vi "Temperature read hard mode 2.vi"() -> ()   [LabVIEW 2020]
panel:
  in  "START/STOP 2":bool
  out "START/STOP":bool
  in  "STOP":bool
  out "Waveform Chart":T1(graph)
  out "WARNING":bool
  in  "Filename":path
  in  "LOW Limit":dbl(slide) scale=0.0..100.0
  in  "C   or   F":bool
  in  "HIGH Limit":dbl(slide) scale=0.0..100.0
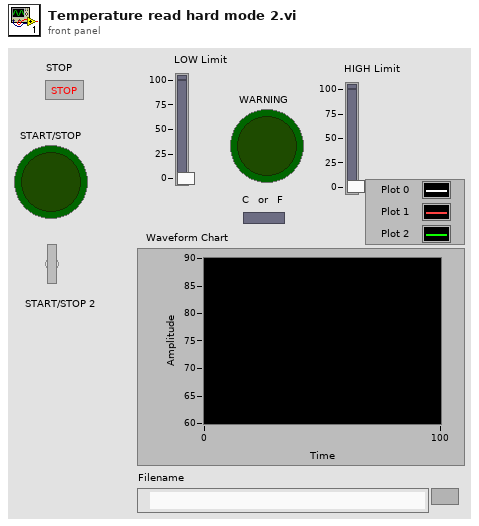
[diagram p1: front panel]
types:
  T1 = cluster{"Temperature (deg F)":dbl, "LOW Limit":dbl, "HIGH Limit":dbl}
  T2 = enum16{"open", "replace", "create", "open or create", "replace or create", "replace or create with confirmation"}
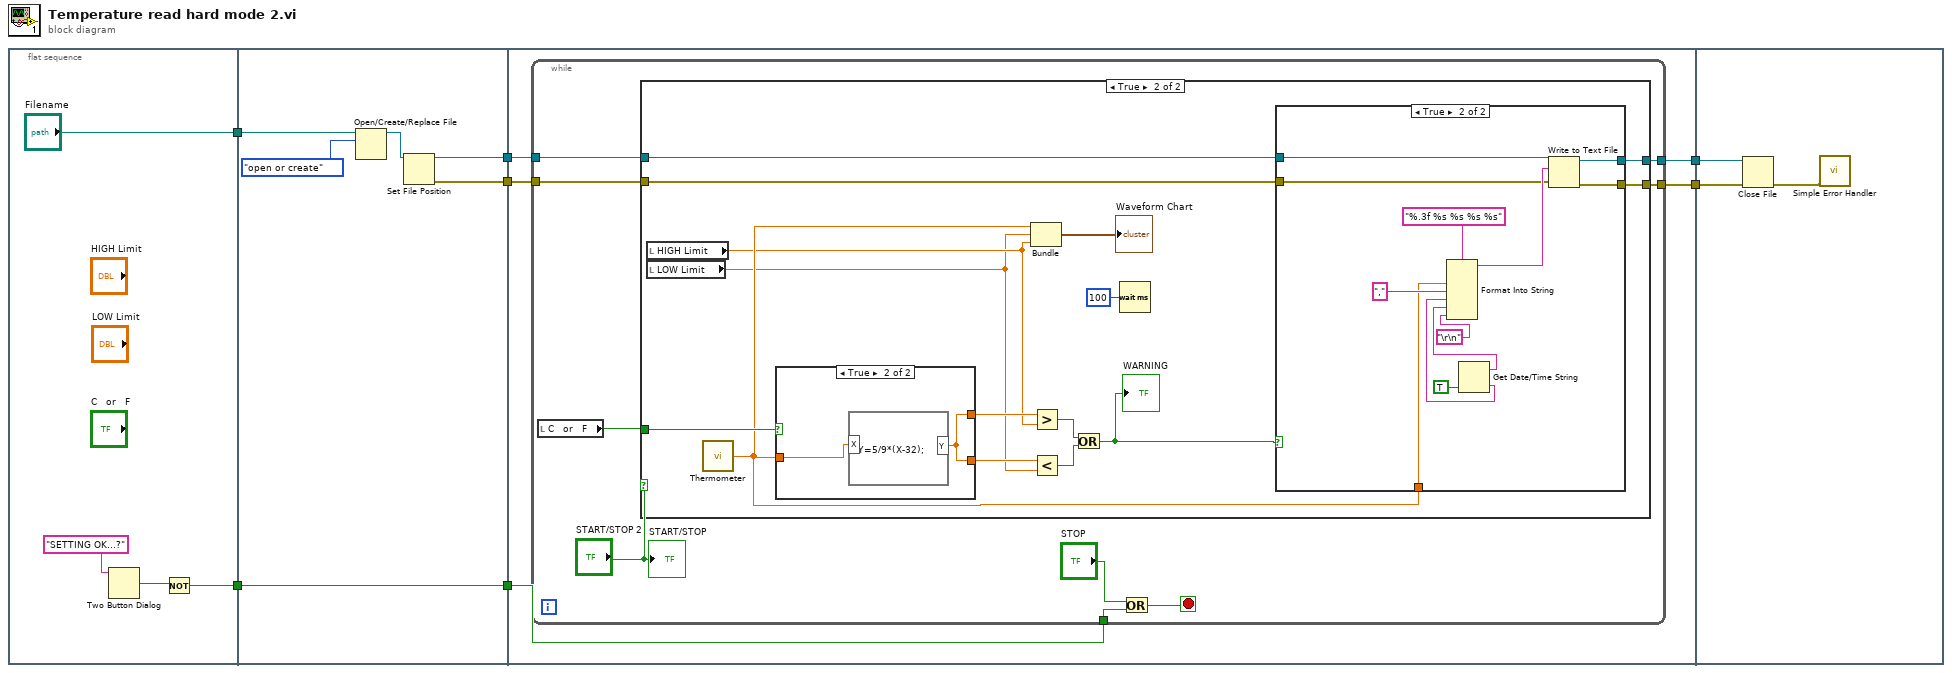
[diagram p0: block diagram]
diagram:
  n1 = flat-sequence {
    tunnel: ["Filename"] -> w7
    tunnel: [w8] -> w6
    tunnel: w7 -> [w17]
    tunnel: [w14] -> w5
    tunnel: w6 -> [w14]
    tunnel: [w13] -> w4
    tunnel: [w12] -> w3
    tunnel: w5 -> [w22]
    tunnel: w4 -> [w21]
    tunnel: w3 -> [w20]
    tunnel: [w19] -> w2
    tunnel: [w18] -> w1
    tunnel: w2 -> [w68]
    tunnel: w1 -> [w67]
    frame #0 {
      n2 = Two Button Dialog(message="SETTING OK...?") -> (T button?=w9:bool)  [unwired: 2 in]
      n3 = Not(x=w9) -> (.not. x?=w8:bool)
    }
    frame #1 {
      n4 = Open/Create/Replace File(file path (use dialog)=w17, operation (0:open)=T2."open or create") -> (refnum out=w15:refnum<file>)  [unwired: 4 in, 2 out]
      n5 = Set File Position(refnum=w15) -> (refnum out=w13:refnum<file>, error out=w12:errorcluster)  [unwired: 3 in]
    }
    frame #2 {
      n6 = while {
        tunnel: w22 -> [w28]
        tunnel: w21 -> [w27]
        tunnel: w20 -> [w26]
        tunnel: [w25] -> w19
        tunnel: [w24] -> w18
        stop <- w29 stop-if-true
        n7 = local read "C   or   F"() -> (w23:bool)
        n8 = case shown="True" "START/STOP 2" {
          tunnel: w23 -> [_ w48]
          tunnel: w27 -> [w33 w39]
          tunnel: w26 -> [w32 w38]
          tunnel: [w33 w37] -> w25
          tunnel: [w32 w36] -> w24
          frame False {
          }
          frame True {
            n9 = local read "HIGH Limit"() -> (w35:dbl)
            n10 = local read "LOW Limit"() -> (w34:dbl)
            n11 = call "Thermometer.vi"() -> ("Temperature (deg F)"=w40:dbl)  [unwired: 1 in]
            n12 = case shown="True" w48 {
              tunnel: w40 -> [w63 w65]
              tunnel: [w63 w64] -> w47
              tunnel: [w63 w64] -> w46
              frame False {
              }
              frame True {
                n13 = formula code="Y=5/9*(X-32);"("X"=w65) -> ("Y"=w64:dbl)
              }
            }
            n14 = Bundle("Temperature (deg F)"=w40, "LOW Limit"=w34, "HIGH Limit"=w35) -> (→"Waveform Chart":T1)  [unwired: 1 in]
            n15 = Greater?(x=w47, y=w35) -> (0:w45:bool)
            n16 = Less?(x=w46, y=w34) -> (x < y?=w44:bool)
            n17 = Or(x=w45, y=w44) -> (x .or. y?=w42:bool)
            "WARNING" <- w42
            n18 = Wait (ms)(milliseconds to wait=u32 100) -> ()  [unwired: 1 out]
            n19 = case shown="True" w42 {
              tunnel: w40 -> [_ w60]
              tunnel: w39 -> [w49 w55]
              tunnel: w38 -> [w50 w54]
              tunnel: [w49 w53] -> w37
              tunnel: [w50 w52] -> w36
              frame False {
              }
              frame True {
                n20 = Get Date/Time String(want seconds? (F)=TRUE) -> (date string=w59:string, time string=w58:string)  [unwired: 2 in]
                n21 = Format Into String(format string="%.3f %s %s %s %s", w60, "," ("input 2"), w58, w59, "\r\n") -> (resulting string=w56:string)  [unwired: 2 in, 1 out]
                n22 = Write to Text File(file (use dialog)=w55, text=w56, error in=w54) -> (refnum out=w53:refnum<file>, error out=w52:errorcluster)  [unwired: 1 in, 1 out]
              }
            }
          }
        }
        n23 = Or(x="STOP", y=w28) -> (x .or. y?=w29:bool)
        "START/STOP" <- "START/STOP 2"
      }
    }
    frame #3 {
      n24 = Close File(refnum=w68, error in=w67) -> (error out=w66:errorcluster)  [unwired: 1 out]
      n25 = call <vilib>:"Simple Error Handler.vi"("error in (no error)"=w66) -> ()  [unwired: 4 in, 5 out]
    }
  }
